vi "Configure Contact Check Measurement.vi"(7 "Resistance Threshold (50 Ohm)":dbl=50.0, 8 "error in (no error)":errorcluster, 9 "Measurement Speed (0: Fast)":i32(ring) items=["Fast", "Medium", "Slow"], 10 "Source Measure Unit Channel (0: Channel A)":i32(ring) items=["Channel A", "Channel B"], 11 "VISA resource name":refnum<visa-resource-name>) -> (0 "error out":errorcluster, 3 "VISA resource name out":refnum<visa-resource-name>)   [LabVIEW 2015, in "Keithley 2600 Series.lvlib"]
doc: "Configures the basic settings of the contact check measurement.\n\n<b>Notes:</b>\n(1) This VI is not available on the models 2604B, 2614B, 2634B.\n(2) To use contact check, the current limit must be at least 1 mA (this allows enough current to flow when performing the test), and the SMU (Source Measure Unit) must not be in High-Z output-off mode."
uses:
  Keithley 2600 Series.lvlib
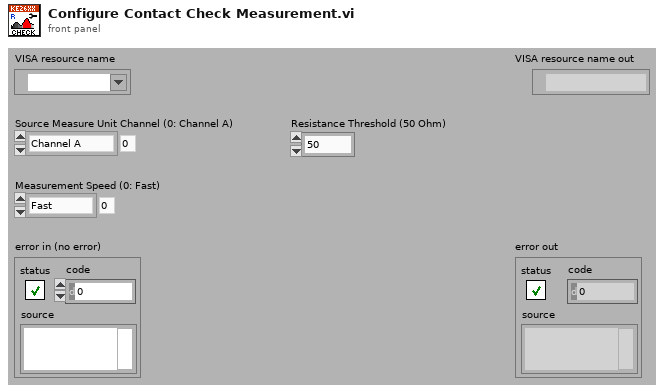
[diagram p1: front panel]
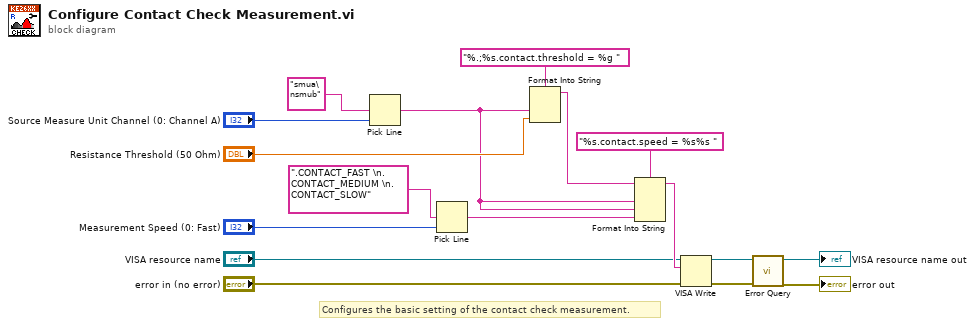
[diagram p0: block diagram]
diagram:
  # "Configures the basic setting of the contact check measurement."
  n1 = Pick Line(multi-line string="smua\nsmub", line index="Source Measure Unit Channel (0: Channel A)") -> (output string=w1:string)  [unwired: 1 in]
  n2 = Pick Line(multi-line string=".CONTACT_FAST \n.CONTACT_MEDIUM \n.CONTACT_SLOW", line index="Measurement Speed (0: Fast)") -> (output string=w2:string)  [unwired: 1 in]
  n3 = Format Into String(format string="%.;%s.contact.threshold = %g ", w1, "Resistance Threshold (50 Ohm)") -> (resulting string=w15:string)  [unwired: 2 in, 1 out]
  n4 = Format Into String(format string="%s.contact.speed = %s%s ", initial string=w15, w1, w1, w2) -> (resulting string=w13:string)  [unwired: 1 in, 1 out]
  n5 = VISA Write(VISA resource name="VISA resource name", write buffer=w13, error in (no error)="error in (no error)") -> (VISA resource name out=w10:refnum<visa-resource-name>, error out=w9:errorcluster)  [unwired: 1 out]
  n6 = call "Error Query.vi"("error in (no error)"=w9, "VISA resource name"=w10) -> ("error out"=→"error out":errorcluster, "VISA resource name out"=→"VISA resource name out":refnum<visa-resource-name>)  [unwired: 6 in, 2 out]
